vi "Actuate.vi"(0 "Dual Cylinder Actuator in":refnum<class "Dual Cylinder Outer Loop Actuator.lvclass">, 5 "FC1 ILC in":refnum<class "ILC.lvclass">, 7 "FC2 ILC in":refnum<class "ILC.lvclass">, 9 "Actuate Settings":T3 {"FC2 Measured Value" format="%.3f"; "Lateral Demand" format="%.3f"; "FC1 Measured Value" format="%.3f"; "Axial Demand" format="%.3f"}, 11 "error in (no error)":errorcluster) -> (4 "Dual Cylinder Actuator out":refnum<class "Dual Cylinder Outer Loop Actuator.lvclass">, 6 "FC1 ILC out":refnum<class "ILC.lvclass">, 8 "FC2 ILC out":refnum<class "ILC.lvclass">, 10 "Actuate Results":T1 {"FC2 Demand" format="%.3f"; "FC1 Demand" format="%.3f"}, 15 "error out":errorcluster)   [LabVIEW 2015, in "Dual Cylinder Outer Loop Actuator.lvclass"]
uses:
  Dual Cylinder Outer Loop Actuator.lvclass
  <userlib>/Common/ILC/ILC/ILC.lvclass
  Typedefs/Actuate Arguments.ctl
  Typedefs/Actuate Results.ctl
  Typedefs/Cylinder Results.ctl
  Dual Cylinder Outer Loop Actuator.lvclass/Dual Cylinder Outer Loop Actuator.ctl
  Actuator Cylinder/Actuator Cylinder/Actuator Cylinder.lvclass
  Typedefs/FAMT Typedefs.lvlib
  Calculators/Actuator To Cylinder Forces/Actuator To Cylinder Forces.lvclass
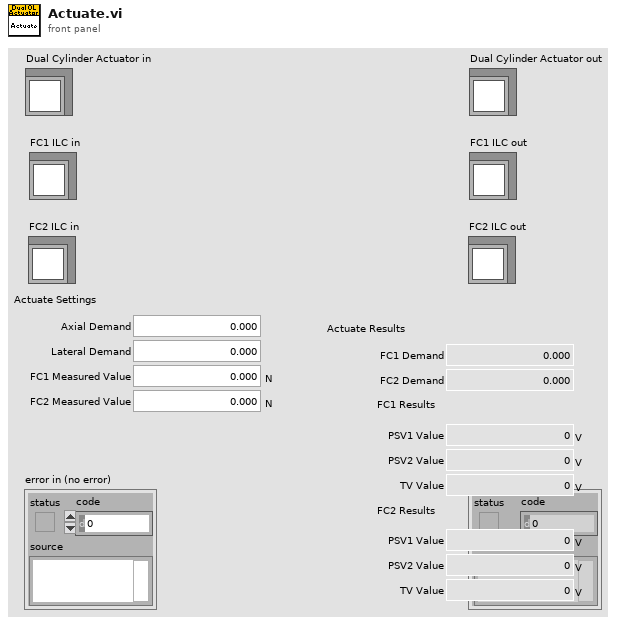
[diagram p1: front panel]
types:
  T1 = typedef "FAMT Typedefs.lvlib/Actuate Results.ctl" = cluster{"FC1 Demand":dbl, "FC2 Demand":dbl, "FC1 Results":T2, "FC2 Results":T2}
  T2 = typedef "FAMT Typedefs.lvlib/Cylinder Results.ctl" = cluster{"PSV1 Value":dbl[unit], "PSV2 Value":dbl[unit], "TV Value":dbl[unit]}
  T3 = typedef "FAMT Typedefs.lvlib/Actuate Arguments.ctl" = cluster{"Axial Demand":dbl, "Lateral Demand":dbl, "FC1 Measured Value":dbl[unit], "FC2 Measured Value":dbl[unit]}
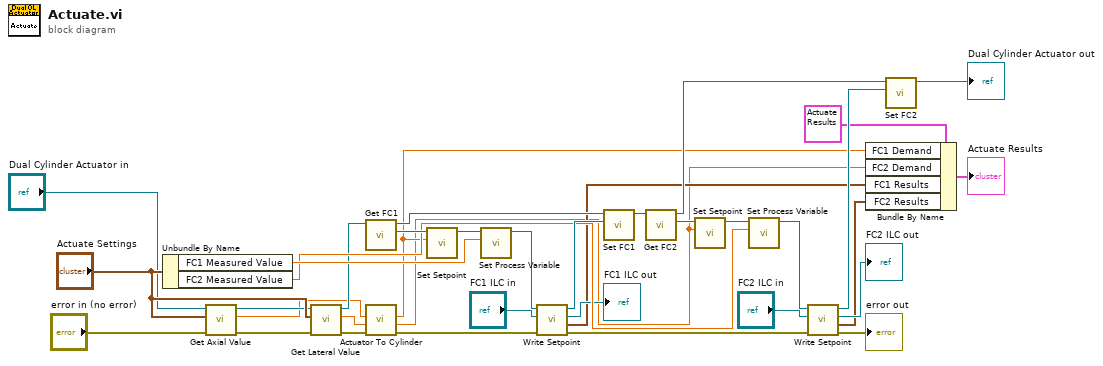
[diagram p0: block diagram]
diagram:
  n1 = Unbundle By Name("Actuate Settings") -> ("FC1 Measured Value"=w21:dbl[unit], "FC2 Measured Value"=w20:dbl[unit])
  n2 = call-dynamic "Get Axial Value.vi"("error in (no error)"="error in (no error)", "Actuate Settings"="Actuate Settings", "Dual Cylinder Outer Loop Actuator in"="Dual Cylinder Actuator in") -> ("error out"=w6:errorcluster, "Axial Control"=w3:dbl[unit], "Dual Cylinder Outer Loop Actuator out"=w9:refnum<class "Dual Cylinder Outer Loop Actuator.lvclass">)  [unwired: 6 in]
  n3 = call-dynamic "Get Lateral Value.vi"("error in (no error)"=w6, "Actuate Settings"="Actuate Settings", "Dual Cylinder Outer Loop Actuator in"=w9) -> ("error out"=w5:errorcluster, "Lateral Control"=w11:dbl[unit], "Dual Cylinder Outer Loop Actuator out"=w8:refnum<class "Dual Cylinder Outer Loop Actuator.lvclass">)  [unwired: 6 in]
  n4 = call "Get FC1.vi"("SingleCylinderActuator in"=w8) -> ("FC1"=w36:refnum<class "Actuator Cylinder.lvclass">, "SingleCylinderActuator out"=w31:refnum<class "Dual Cylinder Outer Loop Actuator.lvclass">)  [unwired: 9 in]
  n5 = call "Actuator To Cylinder.vi"("error in (no error)"=w5, "Lateral Force"=w11, "Axial Force"=w3) -> ("error out"=w4:errorcluster, "FC2 Value"=w1:dbl, "FC1 Value"=w2:dbl)  [unwired: 5 in, 1 out]
  n6 = call-dynamic "Set Setpoint.vi"("Setpoint"=w2, "Actuator Cylinder in"=w36) -> ("Actuator Cylinder out"=w35:refnum<class "Actuator Cylinder.lvclass">)  [unwired: 9 in]
  n7 = call-dynamic "Set Process Variable.vi"("Process Variable"=w21, "Actuator Cylinder in"=w35) -> ("Actuator Cylinder out"=w33:refnum<class "Actuator Cylinder.lvclass">)  [unwired: 9 in]
  n8 = call-dynamic "Write Setpoint.vi"("error in (no error)"=w4, "ILC in"="FC1 ILC in", "Actuator Cylinder in"=w33) -> ("error out"=w28:errorcluster, "Cylinder Results"=w14:T2, "ILC out"=→"FC1 ILC out":refnum<class "ILC.lvclass">, "Actuator Cylinder out"=w32:refnum<class "Actuator Cylinder.lvclass">)  [unwired: 5 in]
  n9 = call "Set FC1.vi"("FC1"=w32, "SingleCylinderActuator in"=w31) -> ("SingleCylinderActuator out"=w30:refnum<class "Dual Cylinder Outer Loop Actuator.lvclass">)  [unwired: 9 in]
  n10 = call "Get FC2.vi"("DualCylinderActuator in"=w30) -> ("FC2"=w25:refnum<class "Actuator Cylinder.lvclass">, "DualCylinderActuator out"=w24:refnum<class "Dual Cylinder Outer Loop Actuator.lvclass">)  [unwired: 9 in]
  n11 = call-dynamic "Set Setpoint.vi"("Setpoint"=w1, "Actuator Cylinder in"=w25) -> ("Actuator Cylinder out"=w26:refnum<class "Actuator Cylinder.lvclass">)  [unwired: 9 in]
  n12 = call-dynamic "Set Process Variable.vi"("Process Variable"=w20, "Actuator Cylinder in"=w26) -> ("Actuator Cylinder out"=w27:refnum<class "Actuator Cylinder.lvclass">)  [unwired: 9 in]
  n13 = call-dynamic "Write Setpoint.vi"("error in (no error)"=w28, "ILC in"="FC2 ILC in", "Actuator Cylinder in"=w27) -> ("error out"=→"error out":errorcluster, "Cylinder Results"=w13:T2, "ILC out"=→"FC2 ILC out":refnum<class "ILC.lvclass">, "Actuator Cylinder out"=w23:refnum<class "Actuator Cylinder.lvclass">)  [unwired: 5 in]
  n14 = Bundle By Name(cluster=T1 {"FC1 Demand"=0.0, "FC2 Demand"=0.0, "FC1 Results"={"PSV1 Value"=0.0, "PSV2 Value"=0.0, "TV Value"=0.0}, "FC2 Results"={"PSV1 Value"=0.0, "PSV2 Value"=0.0, "TV Value"=0.0}} ("Actuate Results"), "FC1 Demand"=w2, "FC2 Demand"=w1, "FC1 Results"=w14, "FC2 Results"=w13) -> (→"Actuate Results":T1)
  n15 = call "Set FC2.vi"("FC2"=w23, "DualCylinderActuator in"=w24) -> ("DualCylinderActuator out"=→"Dual Cylinder Actuator out":refnum<class "Dual Cylinder Outer Loop Actuator.lvclass">)  [unwired: 9 in]
